vi "process_storage.vi"(6 "error in (no error)":errorcluster) -> (0 "error out":errorcluster)   [LabVIEW 2010]
uses:
  typedefs/control_storage_enum.ctl
  typedefs/data_array.ctl
  typedefs/storage_parameters_cluster.ctl
panel:
  out "Last stored package t0":timestamp format="%<%.3X>T"
  out "Filename":path
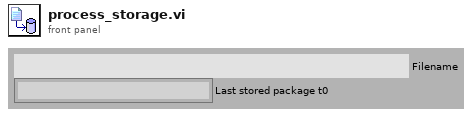
[diagram p1: front panel]
types:
  T1 = typedef "data_array.ctl" = waveform(dbl)[]
  T2 = typedef "control_storage_enum.ctl" = enum16{"Init", "Discard", "Store", "Reset", "Stop", "Quit"}
  T3 = cluster{"Control storage enum":T2, "variant":variant}
  T4 = typedef "storage_parameters_cluster.ctl" = cluster{"Store?":bool, "Path":path, "Basename":string, "Auto-increment?":bool}
  T5 = enum16{"open", "replace", "create", "open or create", "replace or create", "replace or create with confirmation"}
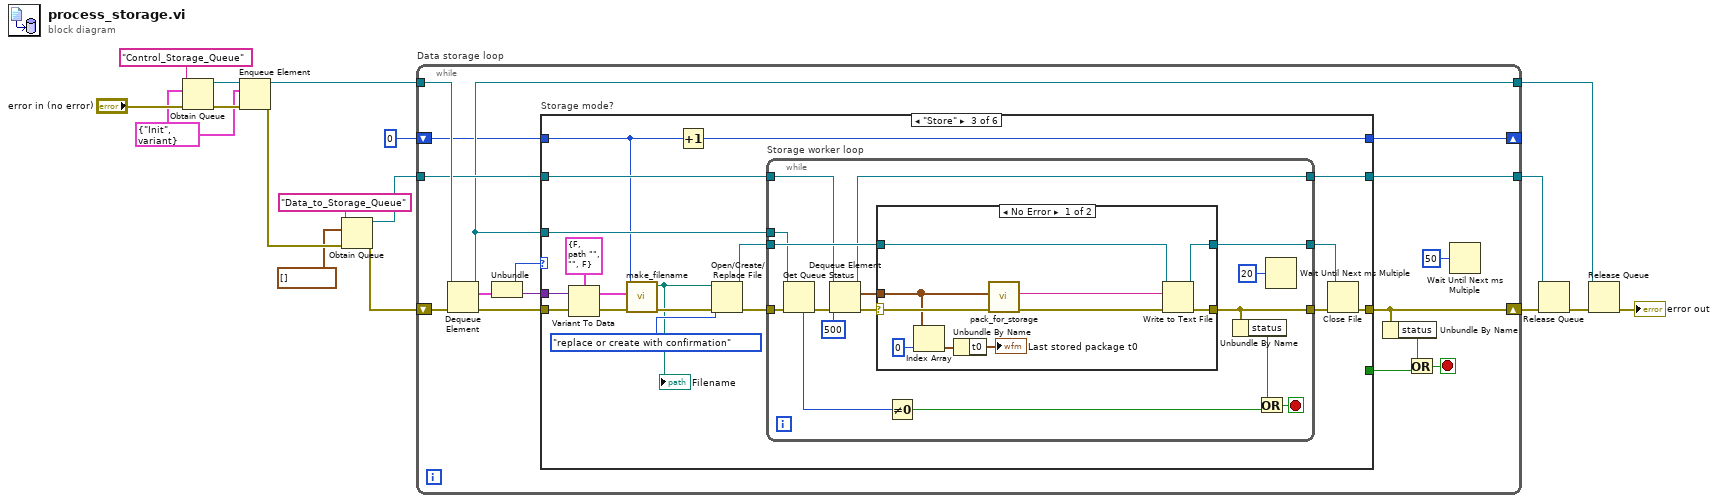
[diagram p0: block diagram]
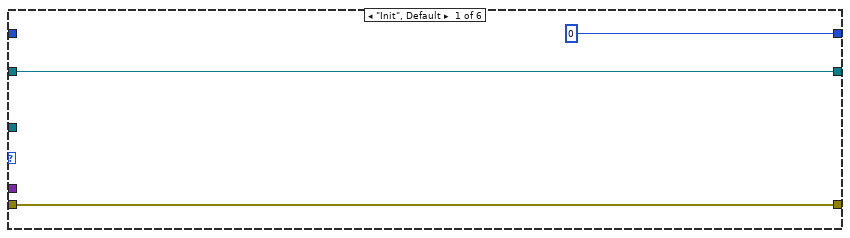
[diagram p2: hidden frame]
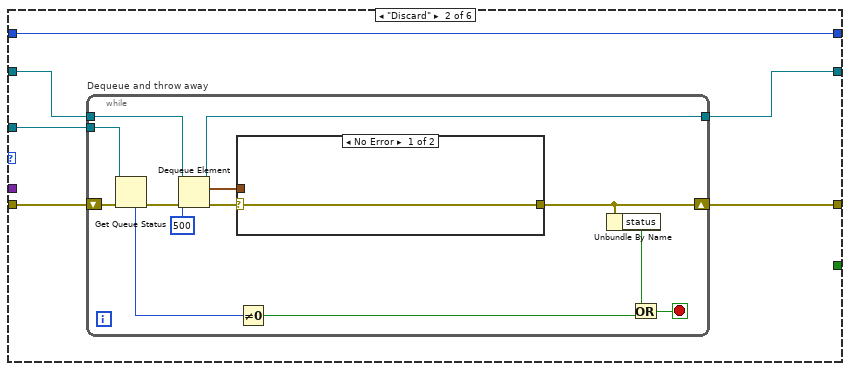
[diagram p3: hidden frame]
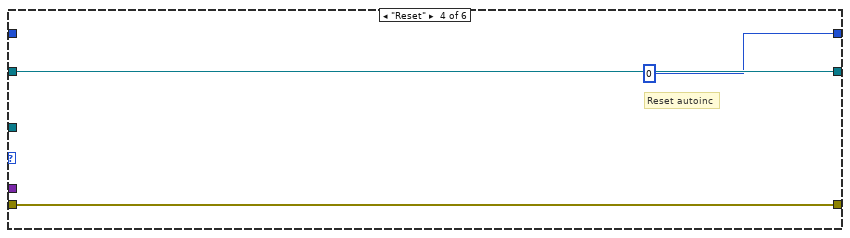
[diagram p6: hidden frame]
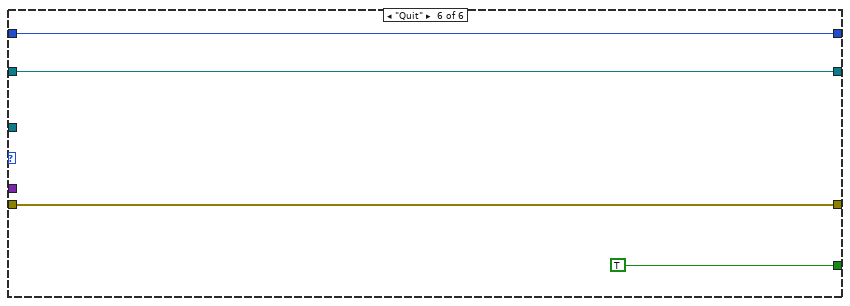
[diagram p8: hidden frame]
diagram:
  w8 = T3 {"Control storage enum"=enum."Init", "variant"=variant}
  n1 = Obtain Queue(name (unnamed)="Control_Storage_Queue", element data type=w8, error in (no error)="error in (no error)") -> (queue out=w11:refnum<queue>, error out=w9:errorcluster)  [unwired: 2 in, 1 out]
  n2 = Enqueue Element(queue=w11, element=w8, error in (no error)=w9) -> (queue out=w10:refnum<queue>, error out=w7:errorcluster)  [unwired: 1 in, 1 out]
  n3 = Obtain Queue(name (unnamed)="Data_to_Storage_Queue", element data type=T1 [] ("Data cluster"), error in (no error)=w7) -> (queue out=w4:refnum<queue>, error out=w3:errorcluster)  [unwired: 2 in, 1 out]
  n4 = while "Data storage loop" {
    shift-right: [w25] -> w6
    shift-left: w3 -> [w31]
    tunnel: w10 -> [w32]
    tunnel: [w21] -> w13
    tunnel: w4 -> [w26]
    tunnel: [w33] -> w12
    shift-right: [w19] -> _
    shift-left: 0 ("Fileno.") -> [w20]
    stop <- w23 stop-if-true
    n5 = Dequeue Element(queue=w32, error in (no error)=w31) -> (queue out=w21:refnum<queue>, element=w30:T3, error out=w27:errorcluster)  [unwired: 1 in, 1 out]
    n6 = Unbundle(w30) -> ("Control storage enum"=w29:T2, "variant"=w28:variant)
    n7 = case "Storage mode?" shown="\"Store\"" w29 {
      tunnel: [w35 w39 w69 w106 w109 w113] -> w33
      tunnel: w28 -> [_ _ w73 _ _ _]
      tunnel: w27 -> [w36 w40 w75 w105 w108 w111]
      tunnel: w26 -> [w35 w42 w72 w106 w109 w113]
      tunnel: [w36 w38 w67 w105 w108 w111] -> w25
      tunnel: [_ _ _ _ _ TRUE] -> w22
      tunnel: w21 -> [_ w41 w71 _ _ _]
      tunnel: w20 -> [_ w37 w60 _ w107 w110]
      tunnel: [0 ("Fileno.") w37 w59 0 ("Fileno.") w107 w110] -> w19
      frame "Init", Default {
      }
      frame "Discard" {
        n8 = while "Dequeue and throw away" {
          tunnel: w42 -> [w49]
          tunnel: w41 -> [w54]
          shift-right: [w44] -> w38
          shift-left: w40 -> [w55]
          tunnel: [w46] -> w39
          stop <- w51 stop-if-true
          n9 = Get Queue Status(queue=w54, error in (no error)=w55) -> (error out=w50:errorcluster, # elements in queue=w53:i32)  [unwired: 1 in, 6 out]
          n10 = Dequeue Element(queue=w49, timeout in ms (-1)=500, error in (no error)=w50) -> (queue out=w46:refnum<queue>, element=w43:T1, error out=w45:errorcluster)  [unwired: 1 out]
          n11 = case shown="No Error" w45 {
            selector: w45 -> [w56 w57]
            tunnel: [w56 w57] -> w44
            tunnel: w43 -> [_ _]
            frame No Error {
            }
            frame Error {
            }
          }
          n12 = Not Equal To 0?(x=w53) -> (x != 0?=w52:bool)
          n13 = Unbundle By Name(w44) -> ("status"=w47:bool)
          n14 = Or(x=w47, y=w52) -> (x .or. y?=w51:bool)
        }
      }
      frame "Store" {
        n15 = Variant To Data(error in=w75, Variant=w73, type=T4 {"Store?"=FALSE, "Path"=path "", "Basename"="", "Auto-increment?"=FALSE} ("Storage parameters")) -> (error out=w63:errorcluster, data=w61:T4)
        n16 = call "make_filename.vi"("error in (no error)"=w63, "Storage parameters"=w61, "Fileno."=w60) -> ("error out"=w62:errorcluster, "Path"=w58:path)  [unwired: 7 in]
        "Filename" <- w58
        n17 = Increment(x=w60) -> (x+1=w59:i32)
        n18 = Open/Create/Replace File(file path (use dialog)=w58, error in=w62, operation (0:open)=T5."replace or create with confirmation") -> (refnum out=w70:refnum<file>, error out=w74:errorcluster)  [unwired: 3 in, 1 out]
        n19 = while "Storage worker loop" {
          tunnel: w72 -> [w79]
          tunnel: [w84] -> w68
          tunnel: w70 -> [w89]
          tunnel: [w88] -> w66
          tunnel: w74 -> [w87]
          tunnel: w71 -> [w85]
          tunnel: [w78] -> w69
          stop <- w80 stop-if-true
          n20 = Get Queue Status(queue=w85, error in (no error)=w87) -> (error out=w86:errorcluster, # elements in queue=w82:i32)  [unwired: 1 in, 6 out]
          n21 = Dequeue Element(queue=w79, timeout in ms (-1)=500, error in (no error)=w86) -> (queue out=w78:refnum<queue>, element=w90:T1, error out=w91:errorcluster)  [unwired: 1 out]
          n22 = case shown="No Error" w91 {
            selector: w91 -> [w98 w103]
            tunnel: [w101 w103] -> w84
            tunnel: w90 -> [w95 _]
            tunnel: w89 -> [w99 w102]
            tunnel: [w100 w102] -> w88
            frame No Error {
              n23 = Index Array(array=w95, index=0) -> (element=w93:waveform(dbl))
              n24 = Unbundle By Name(w93) -> ("t0"=→"Last stored package t0":timestamp)
              n25 = call "pack_for_storage.vi"("error in"=w98, "Data in"=w95) -> ("error out"=w97:errorcluster, "String out"=w96:string)  [unwired: 8 in]
              n26 = Write to Text File(file (use dialog)=w99, text=w96, error in=w97) -> (refnum out=w100:refnum<file>, error out=w101:errorcluster)  [unwired: 1 in, 1 out]
            }
            frame Error {
            }
          }
          n27 = Not Equal To 0?(x=w82) -> (x != 0?=w81:bool)
          n28 = Unbundle By Name(w84) -> ("status"=w83:bool)
          n29 = Or(x=w83, y=w81) -> (x .or. y?=w80:bool)
          n30 = Wait Until Next ms Multiple(millisecond multiple=u32 20) -> ()  [unwired: 1 out]
        }
        n31 = Close File(refnum=w66, error in=w68) -> (error out=w67:errorcluster)  [unwired: 1 out]
      }
      frame "Reset" {
        # "Reset autoinc"
      }
      frame "Stop" {
      }
      frame "Quit" {
      }
    }
    n32 = Unbundle By Name(w25) -> ("status"=w24:bool)
    n33 = Or(x=w24, y=w22) -> (x .or. y?=w23:bool)
    n34 = Wait Until Next ms Multiple(millisecond multiple=u32 50) -> ()  [unwired: 1 out]
  }
  n35 = Release Queue(queue=w12, error in (no error)=w6) -> (error out=w5:errorcluster)  [unwired: 1 in, 2 out]
  n36 = Release Queue(queue=w13, error in (no error)=w5) -> (error out=→"error out":errorcluster)  [unwired: 1 in, 2 out]
